vi "String - Convert UserDefined Date to SQL Date (YYYY-mm-dd).vi"(7 "Date Format (UserDefined)":string, 8 "Error In":errorcluster, 11 "Date String (UserDefined)":string) -> (0 "error out":errorcluster, 2 "time stamp":timestamp, 3 "YYYY-mm-dd":string)   [LabVIEW 2013]
panel:
  # "%Y-%d-%m"
  # "2014-31-01"
  # "2014-01-31"
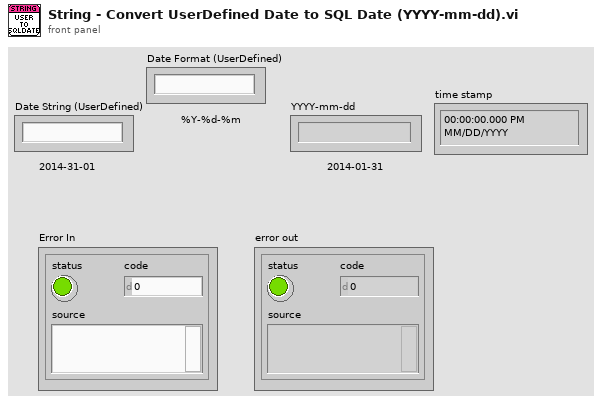
[diagram p1: front panel]
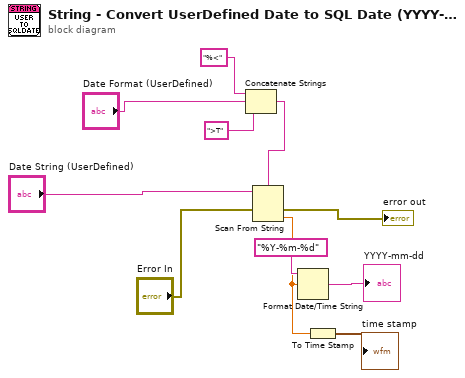
[diagram p0: block diagram]
diagram:
  n1 = Concatenate Strings("%<" ("format string"), "Date Format (UserDefined)", ">T" ("format string")) -> (w4:string)
  n2 = Scan From String(format string=w4, input string="Date String (UserDefined)", error in="Error In") -> (error out=→"error out":errorcluster, output 1=w2:dbl)  [unwired: 2 in, 2 out]
  n3 = Format Date/Time String(time format string (%c)="%Y-%m-%d" ("format string"), seconds (now)=w2) -> (date/time string=→"YYYY-mm-dd":string)  [unwired: 1 in]
  n4 = To Time Stamp(1:w2) -> (0:→"time stamp":timestamp)
